vi "readBlueforsHtml.vi"(7 "Web(T)":bool=TRUE, 8 "Error In":errorcluster, 11 "url":string="http://192.168.0.101:5001/channel/measurement/latest") -> (0 "Error Out":errorcluster, 1 "temperatura":dbl, 2 "chan_nr":i32, 3 "date/time string":string, 4 "STATUS":string, 5 "datoNuevo?":bool=TRUE)   [LabVIEW 2017]
uses:
  datosGraficaBlueforsNumeric.ctl
  <vilib>/httpClient/LabVIEWHTTPClient.lvlib
panel:
  out "Datos":string[](array[string])
  out "Cabecera":string[](array[string])
  out "datos BLUEFORS":T1 {"imz" format="%.3f"; "status_flags" format="%.3f"; "magnitude" format="%.3f"; "reactance" format="%.3f"; "datetime" format="%.3f"; "channel_nr" format="%.3f"; "resistance" format="%.3f"; "timestamp" format="%.3f"; "settings_nr" format="%.3f"; "temperature" format="%.3f"; "angle" format="%.3f"; "status" format="%.3f"; "rez" format="%.3f"}
  out "body":string="{\"rez\": 178.573, \"status\": \"OK\", \"angle\": 90.054, \"temperature\": 4.268984, \"settings_nr\": 17, \"timestamp\": 1655726623.39446, \"resistance\": 178.573, \"channel_nr\": 5, \"datetime\": \"2022-06-20T12:03:55.010794Z\", \"reactance\": -186159.948, \"magnitude\": 178.573, \"status_flags\": [], \"imz\": -0.171}"
  out "headers":string="HTTP/1.1 200 OK\r\nContent-Length: 271\r\nServer: TornadoServer/5.1.1\r\nEtag: \"846106313589bc8d9fa2b11791fa3e2bef692078\"\r\nDate: Wed, 09 Jun 2021 16:16:40 GMT\r\nAccess-Control-Allow-Origin: *\r\nAccess-Control-Allow-Headers: access-control-allow-origin,authorization,content-type\r\nContent-Type: application/json; charset=UTF-8\r\n\r\n"
  # "LEE EL FICHERO TXT ALMACENADO EN EL SERVIDOR WEB\nEXTRAE LOS VALORES ORDENADOS A UNA MATRIZ"
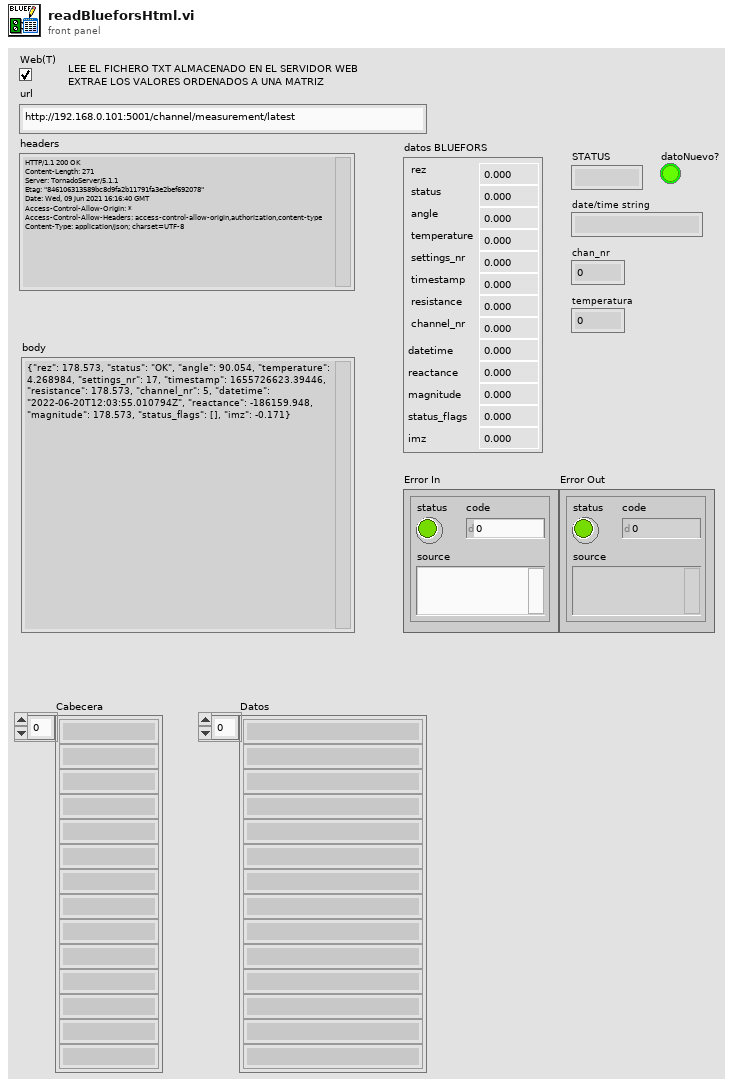
[diagram p1: front panel]
types:
  T1 = typedef "datosGraficaBlueforsNumeric.ctl" = cluster{"rez":dbl, "status":dbl, "angle":dbl, "temperature":dbl, "settings_nr":dbl, "timestamp":dbl, "resistance":dbl, "channel_nr":dbl, "datetime":dbl, "reactance":dbl, "magnitude":dbl, "status_flags":dbl, "imz":dbl}
  T2 = typedef "LabVIEWHTTPClient.lvlib/ClientHandle.ctl" = refnum<k1>
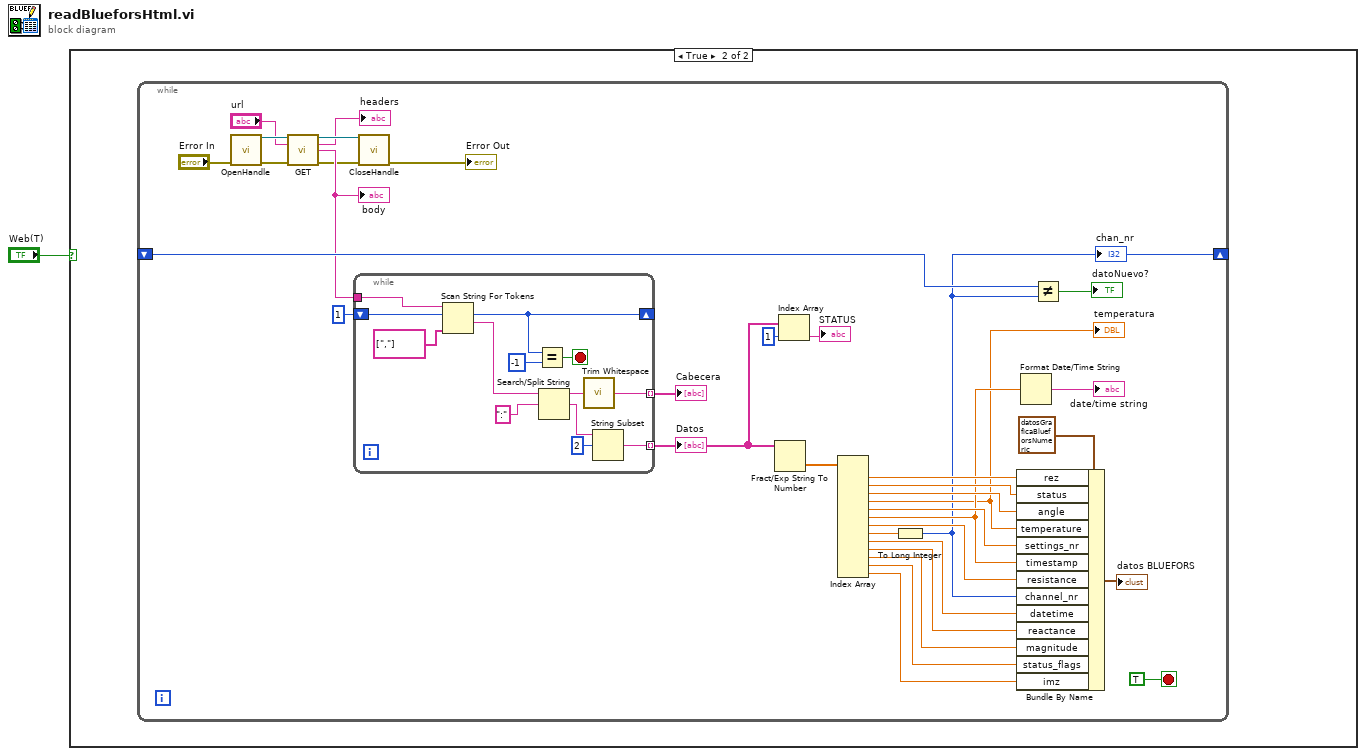
[diagram p0: block diagram]
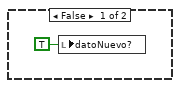
[diagram p2: hidden frame]
diagram:
  n1 = case shown="True" "Web(T)" {
    frame False {
      n2 = local write "datoNuevo?"(TRUE ("datoNuevo?")) -> ()
    }
    frame True {
      n3 = while {
        shift-right: [w3] -> _
        shift-left: _ -> [w31]
        stop <- TRUE stop-if-true
        n4 = call <vilib>:"OpenHandle.vi"("error in (no error)"="Error In") -> ("client handle out"=w26:T2, "error out"=w22:errorcluster)  [unwired: 13 in]
        n5 = call <vilib>:"GET.vi"("client handle"=w26, "url"="url", "error in (no error)"=w22) -> ("client handle out"=w25:T2, "headers"=→"headers":string, "body"=w27:string, "error out"=w23:errorcluster)  [unwired: 9 in]
        "body" <- w27
        n6 = while {
          tunnel: w27 -> [w50]
          shift-right: [w45] -> _
          shift-left: 1 ("offset past token") -> [w48]
          tunnel: [w41] -> w33 mode=indexing
          tunnel: [w39] -> w30 mode=indexing
          stop <- w47 stop-if-true
          n7 = Scan String For Tokens(6:string[] [","] ("operators (none)"), 8:w48, 9:w50) -> (1:w44:string, 2:w45:i32)  [unwired: 3 in, 2 out]
          n8 = Equal?(x=w45, y=-1) -> (x = y?=w47:bool)
          n9 = Search/Split String(string=w44, search string/char (-)=":" ("element")) -> (substring before match=w42:string, match + rest of string=w40:string)  [unwired: 1 in, 1 out]
          n10 = call <vilib>:"Trim Whitespace.vi"("string"=w42) -> ("trimmed string"=w41:string)  [unwired: 1 in]
          n11 = String Subset(string=w40, offset (0)=2) -> (substring=w39:string)  [unwired: 1 in]
        }
        "Cabecera" <- w33
        "Datos" <- w30
        n12 = call <vilib>:"CloseHandle.vi"("client handle"=w25, "error in (no error)"=w23) -> ("error out"=→"Error Out":errorcluster)  [unwired: 13 in]
        n13 = Fract/Exp String To Number(string=w30) -> (number=w32:dbl[])  [unwired: 3 in, 1 out]
        n14 = Index Array(array=w30, index=1) -> (element=→"STATUS":string)
        n15 = Index Array(array=w32) -> (element #1=w19:dbl, element #2=w16:dbl, element #3=w15:dbl, element #4=w4:dbl, element #5=w14:dbl, element #6=w7:dbl, element #7=w13:dbl, element #8=w5:dbl, element #9=w12:dbl, element #10=w11:dbl, element #11=w10:dbl, element #12=w9:dbl, element #13=w8:dbl)  [unwired: 13 in]
        "temperatura" <- w4
        n16 = To Long Integer(number=w5) -> (32bit integer=w3:i32)
        "chan_nr" <- w3
        n17 = Bundle By Name(cluster=T1 {"rez"=93.296, "status"=0.0, "angle"=90.069, "temperature"=25.905019, "settings_nr"=0.0, "timestamp"=0.0, "resistance"=1655898328.20644, "channel_nr"=93.296, "datetime"=0.0, "reactance"=0.0, "magnitude"=-76836.555, "status_flags"=0.0, "imz"=0.0} ("datos BLUEFORS"), "rez"=w19, "status"=w16, "angle"=w15, "temperature"=w4, "settings_nr"=w14, "timestamp"=w7, "resistance"=w13, "channel_nr"=w3, "datetime"=w12, "reactance"=w11, "magnitude"=w10, "status_flags"=w9, "imz"=w8) -> (→"datos BLUEFORS":T1)
        n18 = Format Date/Time String(seconds (now)=w7) -> (date/time string=→"date/time string":string)  [unwired: 2 in]
        n19 = Not Equal?(x=w31, y=w3) -> (x != y?=→"datoNuevo?":bool)
      }
    }
  }
